vi "2D Polynomial Evaluation.vi"(2 "Coefficients: a":dbl[](array[numeric]) format="%0.2f", 3 "X":dbl[][](array[numeric]) format="%0.2f") -> (0 "error":i32, 1 "Y":dbl[][](array[numeric]) format="%0.2f")   [LabVIEW 2014, in "NI_AALBase.lvlib"]
doc: "LabVIEW no longer supports this VI. Use the Polynomial Evaluation VI instead.\nThis VI performs a polynomial evaluation of the 2D input array <b>X</b> using <b>Coefficients: a</b>."
uses:
  NI_AALBase.lvlib
  lvanlys.dll
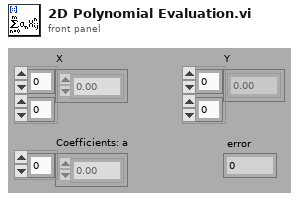
[diagram p1: front panel]
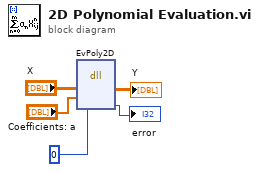
[diagram p0: block diagram]
diagram:
  n1 = dll-call lib="C:/Program Files (x86)/National Instruments/LabVIEW 2014/resource/lvanlys.*" fn="EvPoly2D"("X"="X", "Coefficients: a"="Coefficients: a", 0) -> ("X"=→"Y":dbl[][], →"error":i32)  [unwired: 5 in, 2 out]
